vi "Register Event.vi"(8 "error in (no error)":errorcluster) -> (0 "error out":errorcluster, 3 "Event Registration Refnum":refnum<event-registration>)   [LabVIEW 2016, in "System.lvlib"]
uses:
  System.lvlib
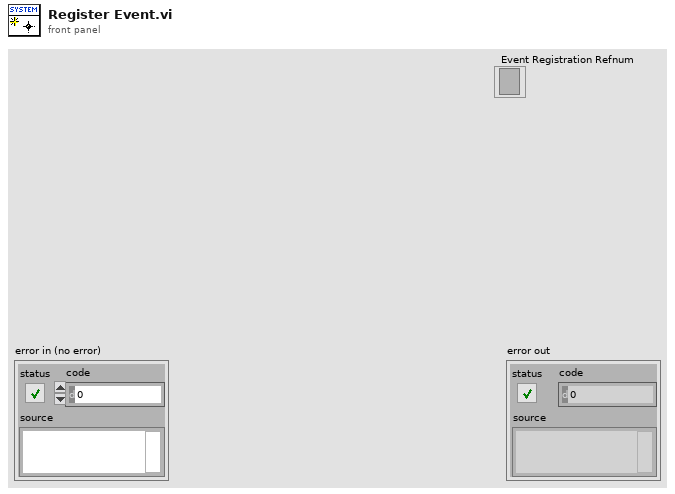
[diagram p1: front panel]
types:
  T1 = typedef "System.lvlib/Control_User Event.ctl" = cluster{"Stop":refnum<user-event>, "Error":refnum<user-event>}
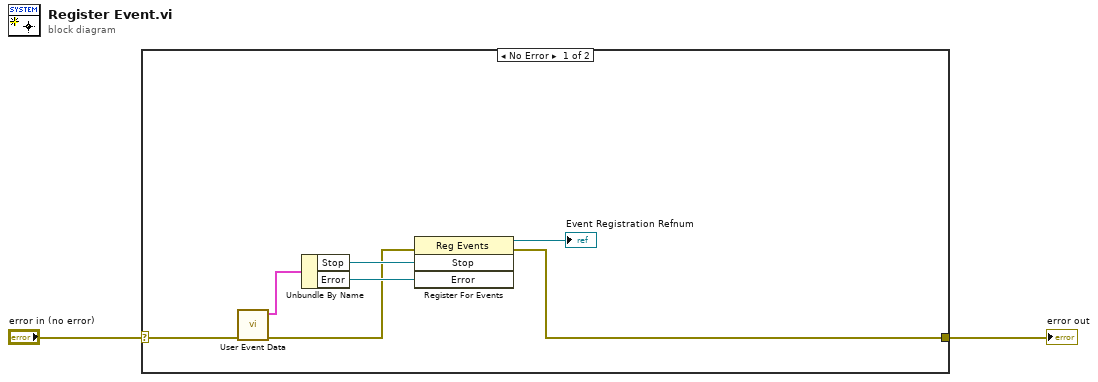
[diagram p0: block diagram]
diagram:
  n1 = case shown="No Error" "error in (no error)" {
    selector: "error in (no error)" -> [w9 w10]
    tunnel: [w4 w10] -> w1
    frame No Error {
      n2 = call "User Event Data.vi"("error in (no error)"=w9) -> ("error out"=w5:errorcluster, "User Event Data"=w8:T1)  [unwired: 9 in]
      n3 = Unbundle By Name(w8) -> ("Stop"=w7:refnum<user-event>, "Error"=w6:refnum<user-event>)
      n4 = register-events(error in=w5, w7, w6) -> (reference out=→"Event Registration Refnum":refnum<event-registration>, error out=w4:errorcluster)  [unwired: 1 in]
    }
    frame Error {
    }
  }
  "error out" <- w1
